vi "ReadModelFile.vi"() -> (0 "error out":errorcluster, 3 "out":string[][](array[string]), 5 "Model":string)   [LabVIEW 2013]
uses:
  SubVi/Global constant.vi
panel:
  in  "Model_N":u16(ring) caption="Model" items=["demo", "demo1", "demo2", "demo3", "demo3_2"]
  in  "OK":bool
  in  "Model":u16(ring) items=["57618362", "57640502", "57640519", "", "", ""]
  in  "Error In":errorcluster
  out "Error Out":errorcluster
  out "ModelList":string[](array[string])
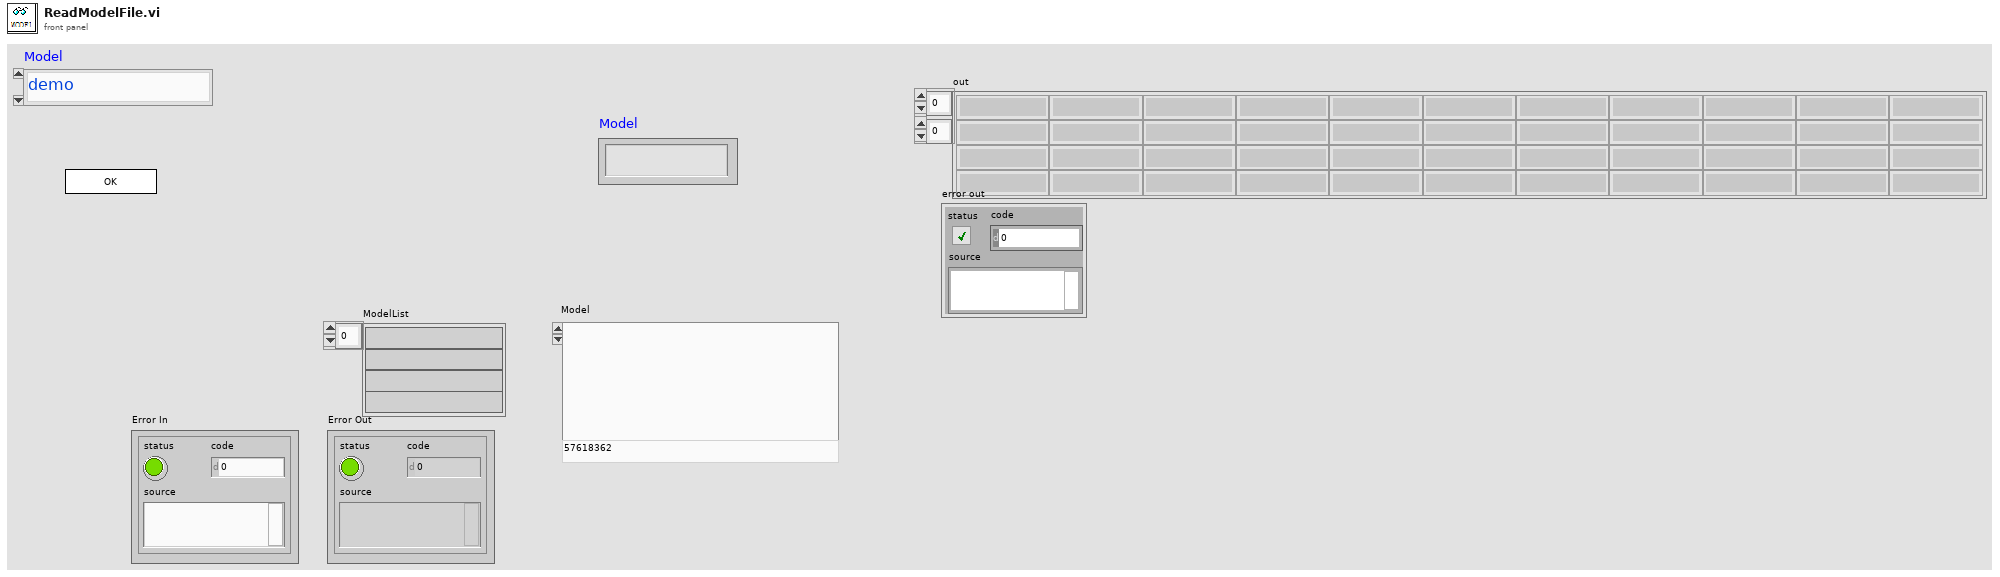
[diagram p1: front panel]
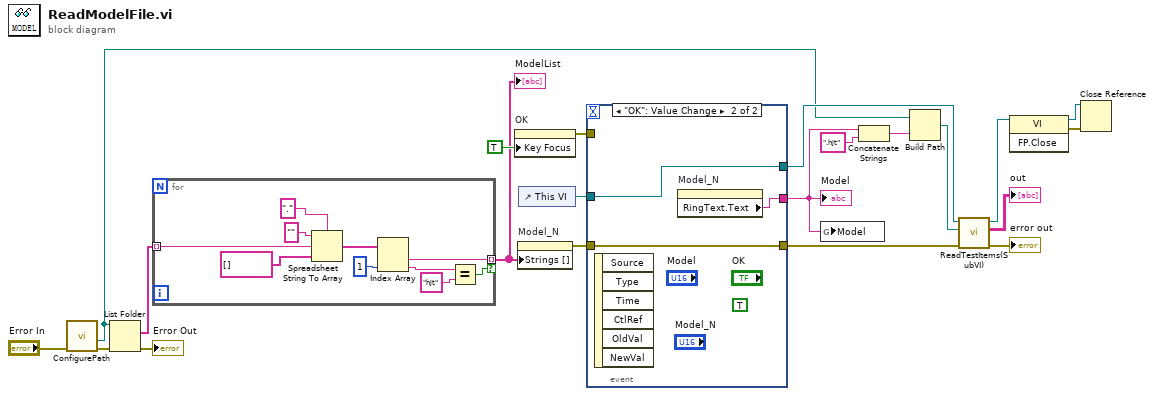
[diagram p0: block diagram]
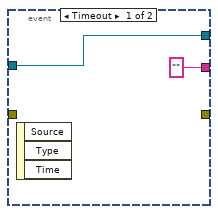
[diagram p2: hidden frame]
diagram:
  n1 = call "ConfigurePath.vi"("Error In"="Error In") -> ("Error Out"=w12:errorcluster, "Folderpath"=w6:path)  [unwired: 7 in, 2 out]
  n2 = List Folder(path=w6, error in=w12) -> (filenames=w21:string[], error out=→"Error Out":errorcluster)  [unwired: 2 in, 2 out]
  n3 = for {
    tunnel: w21 -> [w31] mode=indexing
    tunnel: [w23] -> w11 mode=indexing if=w22
    n4 = Spreadsheet String To Array(delimiter (Tab)=".", format string="", spreadsheet string=w31, array type (2D Dbl)=string[] []) -> (array=w27:string[])
    n5 = Index Array(array=w27, index #2=1 ("index")) -> (element #1=w23:string, element #2=w25:string)  [unwired: 1 in]
    n6 = Equal?(x=w25, y="hjt") -> (x = y?=w22:bool)
  }
  "ModelList" <- w11
  n7 = property on="OK" class="Bool"("Key Focus"=TRUE) -> (error out=w17:errorcluster)  [unwired: 2 in, 1 out]
  n8 = property on="Model_N" class="Ring (严格)"("Strings []"=w11) -> (error out=w14:errorcluster)  [unwired: 2 in, 1 out]
  n9 = control-ref of="This VI"() -> (w18:refnum<vi>)
  n10 = event shown="[1] \"OK\": Value Change" {
    selector: _ -> [_ _]
    dyn-events: _ -> [_ _]
    timeout: _ -> [_ _]
    tunnel: ["" ("Model") w35] -> w5
    tunnel: w14 -> [_ w34]
    tunnel: [w32 w36] -> w9
    tunnel: w18 -> [w32 w36]
    tunnel: w17 -> [_ _]
    tunnel: [_ w34] -> w10
    event Timeout {
      n11 = event-data() -> ()  [unwired: 1 in, 3 out]
    }
    event "OK": Value Change {
      (unwired) TRUE
      n12 = event-data() -> ()  [unwired: 1 in, 6 out]
      n13 = property on="Model_N" class="Ring (严格)"() -> ("RingText.Text"=w35:string)  [unwired: 2 in, 2 out]
    }
  }
  "Model" <- w5
  n14 = global write "Global constant.vi" "Model"(w5) -> ()
  n15 = Concatenate Strings(w5, ".hjt" ("string")) -> (w4:string)
  n16 = Build Path(base path=w6, name or relative path=w4) -> (appended path=w7:path)
  n17 = call "ReadTestItems(SubVI).vi"("error in (no error)"=w10, "Model path"=w7, "VI in"=w9) -> ("error out"=→"error out":errorcluster, "items out"=→"out":string[][], "VI out"=w8:refnum<vi>)  [unwired: 6 in]
  n18 = invoke class="VI" method="FP.Close"(reference=w8) -> (reference out=w19:refnum<vi>, error out=w15:errorcluster)  [unwired: 2 in, 1 out]
  n19 = Close Reference(reference=w19, error in (no error)=w15) -> ()  [unwired: 1 out]
